vi "flow-builder-proc-start.vi"(7 "Step Label":string, 10 "Start(T) / Stop(F)":bool=TRUE, 11 "Proc Name":string) -> (0 "Error":errorcluster, 3 "Step Element":T1)   [LabVIEW 2024]
uses:
  controls/UiStepBuilder.ctl
  controls/type.step-builder.ctl
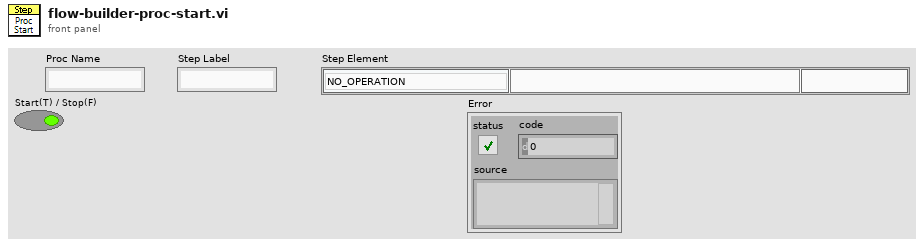
[diagram p1: front panel]
types:
  T1 = typedef "UiStepBuilder.ctl" = cluster{"Step Function":T2, "ParamString":string, "Step Label":string}
  T2 = typedef "type.step-builder.ctl" = enum16{"NO_OPERATION", "DELAY-JUMP", "DELAY", "JUMP", "COMPLETE", "SCHEDULER", "IRR-CHECK", "UNIT-CHECK", "UNIT-SAMPLE", "UNIT-DOSE", "LOG-REPORT", "LOG-MESSAGE", "IO-READ", "IO-READ-MANY", "IO-WRITE", "IO-COMPARE-OUT", "IO-COMPARE-IN", "PROC-START", "PROC-STOP", "PROC-LOAD", "PROC-IS-COMPLETED", "RECORD-MOVE", "GET-RH", "GET-UV", "GET-WD", "GET-WS", "OCS-CHECK", "OCS-RECORD"}
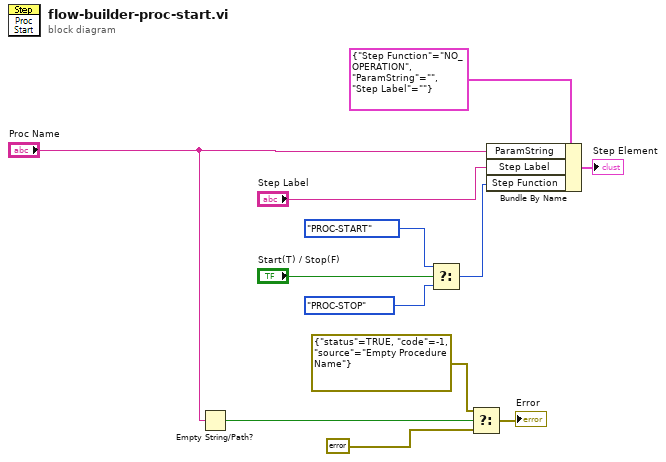
[diagram p0: block diagram]
diagram:
  n1 = Empty String/Path?(string/path="Proc Name") -> (empty?=w4:bool)
  n2 = Select(t=type.step-builder."PROC-START" ("Step Function"), s="Start(T) / Stop(F)", f=type.step-builder."PROC-STOP" ("Step Function")) -> (s? t:f=w6:T2)
  n3 = Select(t=errorcluster {"status"=TRUE, "code"=-1, "source"="Empty Procedure Name"} ("error constant"), s=w4, f=errorcluster {"status"=FALSE, "code"=0, "source"=""} ("error constant")) -> (s? t:f=→"Error":errorcluster)
  n4 = Bundle By Name(cluster=T1 {"Step Function"=enum."NO_OPERATION", "ParamString"="", "Step Label"=""} ("FlowModeConstant 2"), "ParamString"="Proc Name", "Step Label"="Step Label", "Step Function"=w6) -> (→"Step Element":T1)
